vi "RecordGPS.vi"(7 "RecordGPS-Data":bool, 10 "GPS_DataLog":string, 11 "MultiWii Data Cluster 2":refnum<vi>) -> (2 "GPS_DataLogOut":string)   [LabVIEW 2017]
uses:
  IMU_Functions/IMU_Data_Cluster.ctl
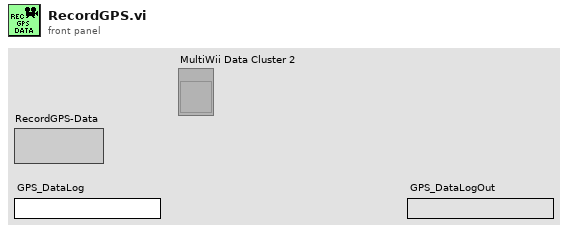
[diagram p1: front panel]
types:
  T1 = typedef "IMU_Data_Cluster.ctl" = cluster{"Firmware Revision":string, "Multitype Name":string, "Cycle Time":u16, "I²C Error Count":u16, "ACC present":bool, "Baro present":bool, "Mag Present":bool, "GPS present":bool, "Sonar present":bool, "Acc X axis (Roll)":dbl, "Acc Y axis (Pitch)":dbl, "Acc Z axis (Yaw)":dbl, "Gyro X axis (Roll)":dbl, "Gyro Y axis (Pitch)":dbl, "Gyro Z axis (Yaw)":dbl, "Mag X axis (Roll)":dbl, "Mag Y axis (Pitch)":dbl, "Mag Z axis (Yaw)":dbl, "X angle (Roll)":dbl, "Y angle (Pitch)":dbl, "Heading [°]":dbl, "Altitude [m]":dbl, "Vario":dbl, "GPS_Fix":u8, "GPS_NumSat":u8, "GPS_coord[LAT]":dbl, "GPS_coord[LON]":dbl, "GPS_Altitude":dbl, "GPS_Speed over Ground":dbl, "GPS_Ground Course":dbl, "Baro P [mbara]":dbl, "Baro T [°C]":dbl, "Altitude abs [m]":dbl}
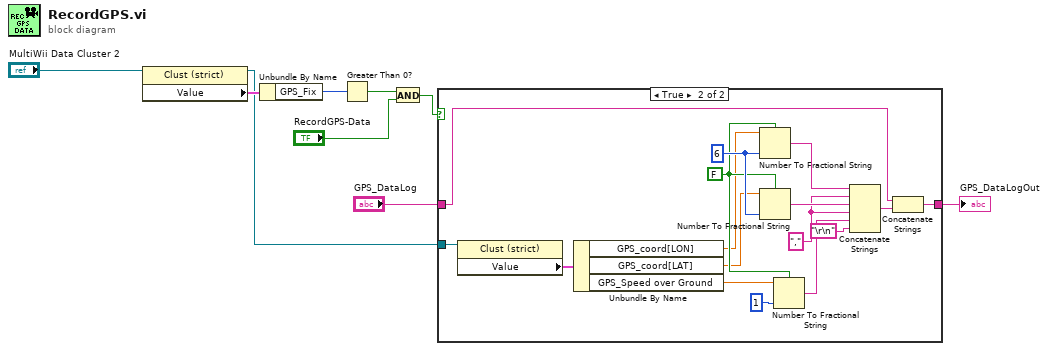
[diagram p0: block diagram]
diagram:
  n1 = property class="Clust (strict)"(reference="MultiWii Data Cluster 2") -> (reference out=w1:refnum<vi>, "Value"=w2:T1)  [unwired: 1 in, 1 out]
  n2 = Unbundle By Name(w2) -> ("GPS_Fix"=w7:u8)
  n3 = Greater Than 0?(x=w7) -> (x > 0?=w6:bool)
  n4 = And(x=w6, y="RecordGPS-Data") -> (x .and. y?=w4:bool)
  n5 = case shown="True" w4 {
    tunnel: "GPS_DataLog" -> [w10 w18]
    tunnel: [w10 w13] -> w8
    tunnel: w1 -> [_ w11]
    frame False {
    }
    frame True {
      w21 = "," ("String")
      w25 = FALSE ("Systemdezimalzeichen verwenden (T)")
      w26 = i16 6 ("Genauigkeit (6)")
      n6 = property class="Clust (strict)"(reference=w11) -> ("Value"=w12:T1)  [unwired: 1 in, 2 out]
      n7 = Unbundle By Name(w12) -> ("GPS_coord[LON]"=w16:dbl, "GPS_coord[LAT]"=w15:dbl, "GPS_Speed over Ground"=w14:dbl)
      n8 = Number To Fractional String(use system decimal point (T)=w25, number=w16, precision (6)=w26) -> (F-format string=w23:string)  [unwired: 1 in]
      n9 = Number To Fractional String(use system decimal point (T)=w25, number=w15, precision (6)=w26) -> (F-format string=w22:string)  [unwired: 1 in]
      n10 = Number To Fractional String(use system decimal point (T)=w25, number=w14, precision (6)=i16 1 ("Genauigkeit (6)")) -> (F-format string=w20:string)  [unwired: 1 in]
      n11 = Concatenate Strings(w23, w21, w22, w21, w20, "\r\n") -> (w17:string)
      n12 = Concatenate Strings(w18, w17) -> (w13:string)
    }
  }
  "GPS_DataLogOut" <- w8
